vi "remoteControlDistance.vi"() -> ()   [LabVIEW 2019]
uses:
  <vilib>/ReMiSYS/ReMiSYS_WSCbot-XS/SubVI/XS_F710.ctl
  <vilib>/ReMiSYS/ReMiSYS_WSCbot-XS/SubVI/XS_stick.ctl
  <vilib>/ReMiSYS/ReMiSYS_WSCbot-XS/SubVI/XS_gamepadF710.lvclass
  <vilib>/Platform/TimedLoop/XDataNode/timing_clust.ctl
  <vilib>/Platform/TimedLoop/XDataNode/nitl_modes.ctl
  <vilib>/Platform/TimedLoop/XDataNode/wakeup.ctl
  <vilib>/platform/TimedLoop/XDataNode/XDataNode.xnode
  <vilib>/Platform/TimedLoop/XDataNode/XDNodeRunTimeDep.lvlib
  WSCbot_V3_Toolkit.lvlibp
panel:
  in  "Correction_distance(V)":dbl=1.5
  out "buttom array":bool[](array[boolean])
  out "Car move (cm)":dbl=-108.003392325
  out "Wheel move (cm)":dbl[](array[numeric])=[329.0260716, 275.9108976, 491.92183620000003, 545.0287023]
  out "F710 button info.leftStick":bool
  out "F710 button info.B":bool
  out "F710 button info.X":bool
  out "F710 button info.A":bool
  out "F710 button info.Y":bool
  out "F710 button info.RB":bool
  out "F710 button info.LB":bool
  out "ini":bool=TRUE
  out "reset":bool
  out "speed":dbl=800.0
  out "Error Out":errorcluster={"status"=FALSE, "code"=1073676418, "source"="VISA Close in XS_usbRawData (SubVI).vi:4400002->XS_gamepadF710.lvlib:XS_gamepadF710.lvclass:XS_grab.vi:4580001->remoteControlDistance.vi"}
  in  "Stop Button":bool
  in  "error in (no error)":errorcluster
  in  "INPUT S/N":string="U16N121E"
  in  "VISA resource name":refnum<visa-resource-name>="USB0::0x046D::0xC21F::145C9E1C::RAW"
  out "Stop Output":bool=TRUE
  out "StepmotorTarget(mm)":dbl=0.2
  out "AxisPosition":dbl
  out "SpeedArray":dbl[](array[numeric])
  out "F710":T1={"RT"=0, "LT"=0, "RightStick"=[{"X"=0.0, "Y"=1.0}], "LeftStick"=[{"X"=3.0, "Y"=0.0}], "Axis info"={"Left x-Axis"=3, "Left y-Axis"=0, "Right x-Axis"=0, "Righ y-Axis"=1, "LT"=0, "RT"=0}, "F710 button info"={"RB"=FALSE, "LB"=FALSE, "rightStick"=FALSE, "leftStick"=FALSE, "start"=FALSE, "back"=FALSE, "right"=FALSE, "left"=FALSE, "down"=FALSE, "up"=FALSE, "Y"=FALSE, "X"=FALSE, "B"=FALSE, "A"=FALSE, "LogiB"=FALSE}}
  in  "maxSpeed":dbl=800.0 format="%#_13g"
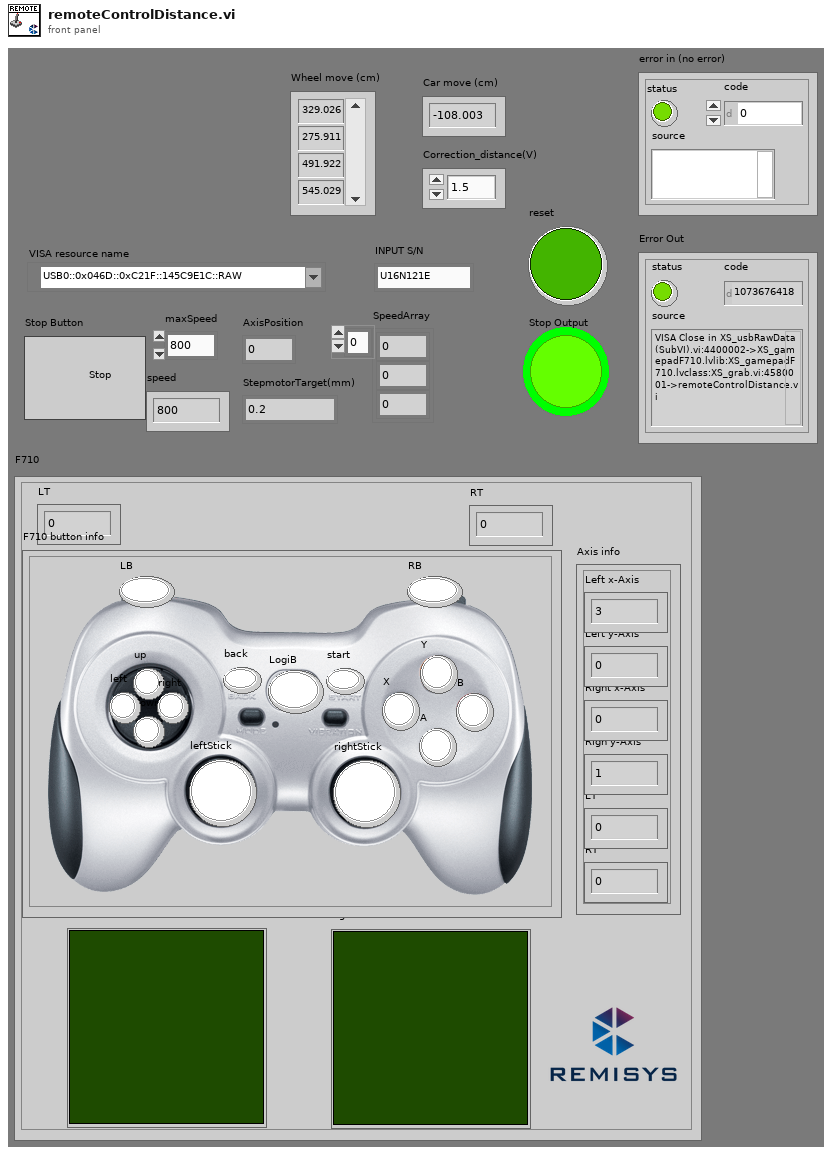
[diagram p1: front panel]
types:
  T1 = typedef "XS_F710.ctl" = cluster{"RT":u8, "LT":u8, "RightStick":T2, "LeftStick":T2, "Axis info":cluster{"Left x-Axis":i8, "Left y-Axis":i8, "Right x-Axis":i8, "Righ y-Axis":i8, "LT":u8, "RT":u8}, "F710 button info":cluster{"RB":bool, "LB":bool, "rightStick":bool, "leftStick":bool, "start":bool, "back":bool, "right":bool, "left":bool, "down":bool, "up":bool, "Y":bool, "X":bool, "B":bool, "A":bool, "LogiB":bool}}
  T2 = typedef "XS_stick.ctl" = cluster{"X":dbl, "Y":dbl}[]
  T3 = typedef "XDNodeRunTimeDep.lvlib/timing_clust.ctl" = cluster{"Expected End [f-1]":u64, "Actual End [f-1]":u64, "Finished Late? [f-1]":bool, "Expected End [i-1]":u64, "Actual End [i-1]":u64, "Finished Late? [i-1]":bool, "Expected Start [i]":u64, "Actual Start [i]":u64, "Expected Start [f]":u64, "Actual Start [f]":u64, "Source Name":string, "Structure Name":string, "Period":i64, "Deadline":i64, "Offset":i64, "Start":i64, "Priority":i32, "Timeout":i32, "Mode":T4, "Wakeup Reason":T5, "Error":errorcluster, "Source Type":string, "Secondary Source Type":string, "Global End Time":u64, "Global Start Time":u64, "Frame Duration":u64, "Iteration Duration":u64, "Assigned CPU":i32, "I/O Scan Engine Mode":u32}
  T4 = typedef "XDNodeRunTimeDep.lvlib/nitl_modes.ctl" = enum32{"No Change", "Process missed periods, maintain original phase", "Discard missed periods, maintain original phase", "Process missed periods, ignore original phase", "Discard missed periods, ignore original phase"}
  T5 = typedef "XDNodeRunTimeDep.lvlib/wakeup.ctl" = enum32{"Normal", "Aborted", "Asynchronous wakeup", "Timing source error", "Timed loop error", "Timeout"}
  T6 = enum16{"Right_up", "Right_down", "Left_down", "Left_up", "left", "right", "up", "down"}
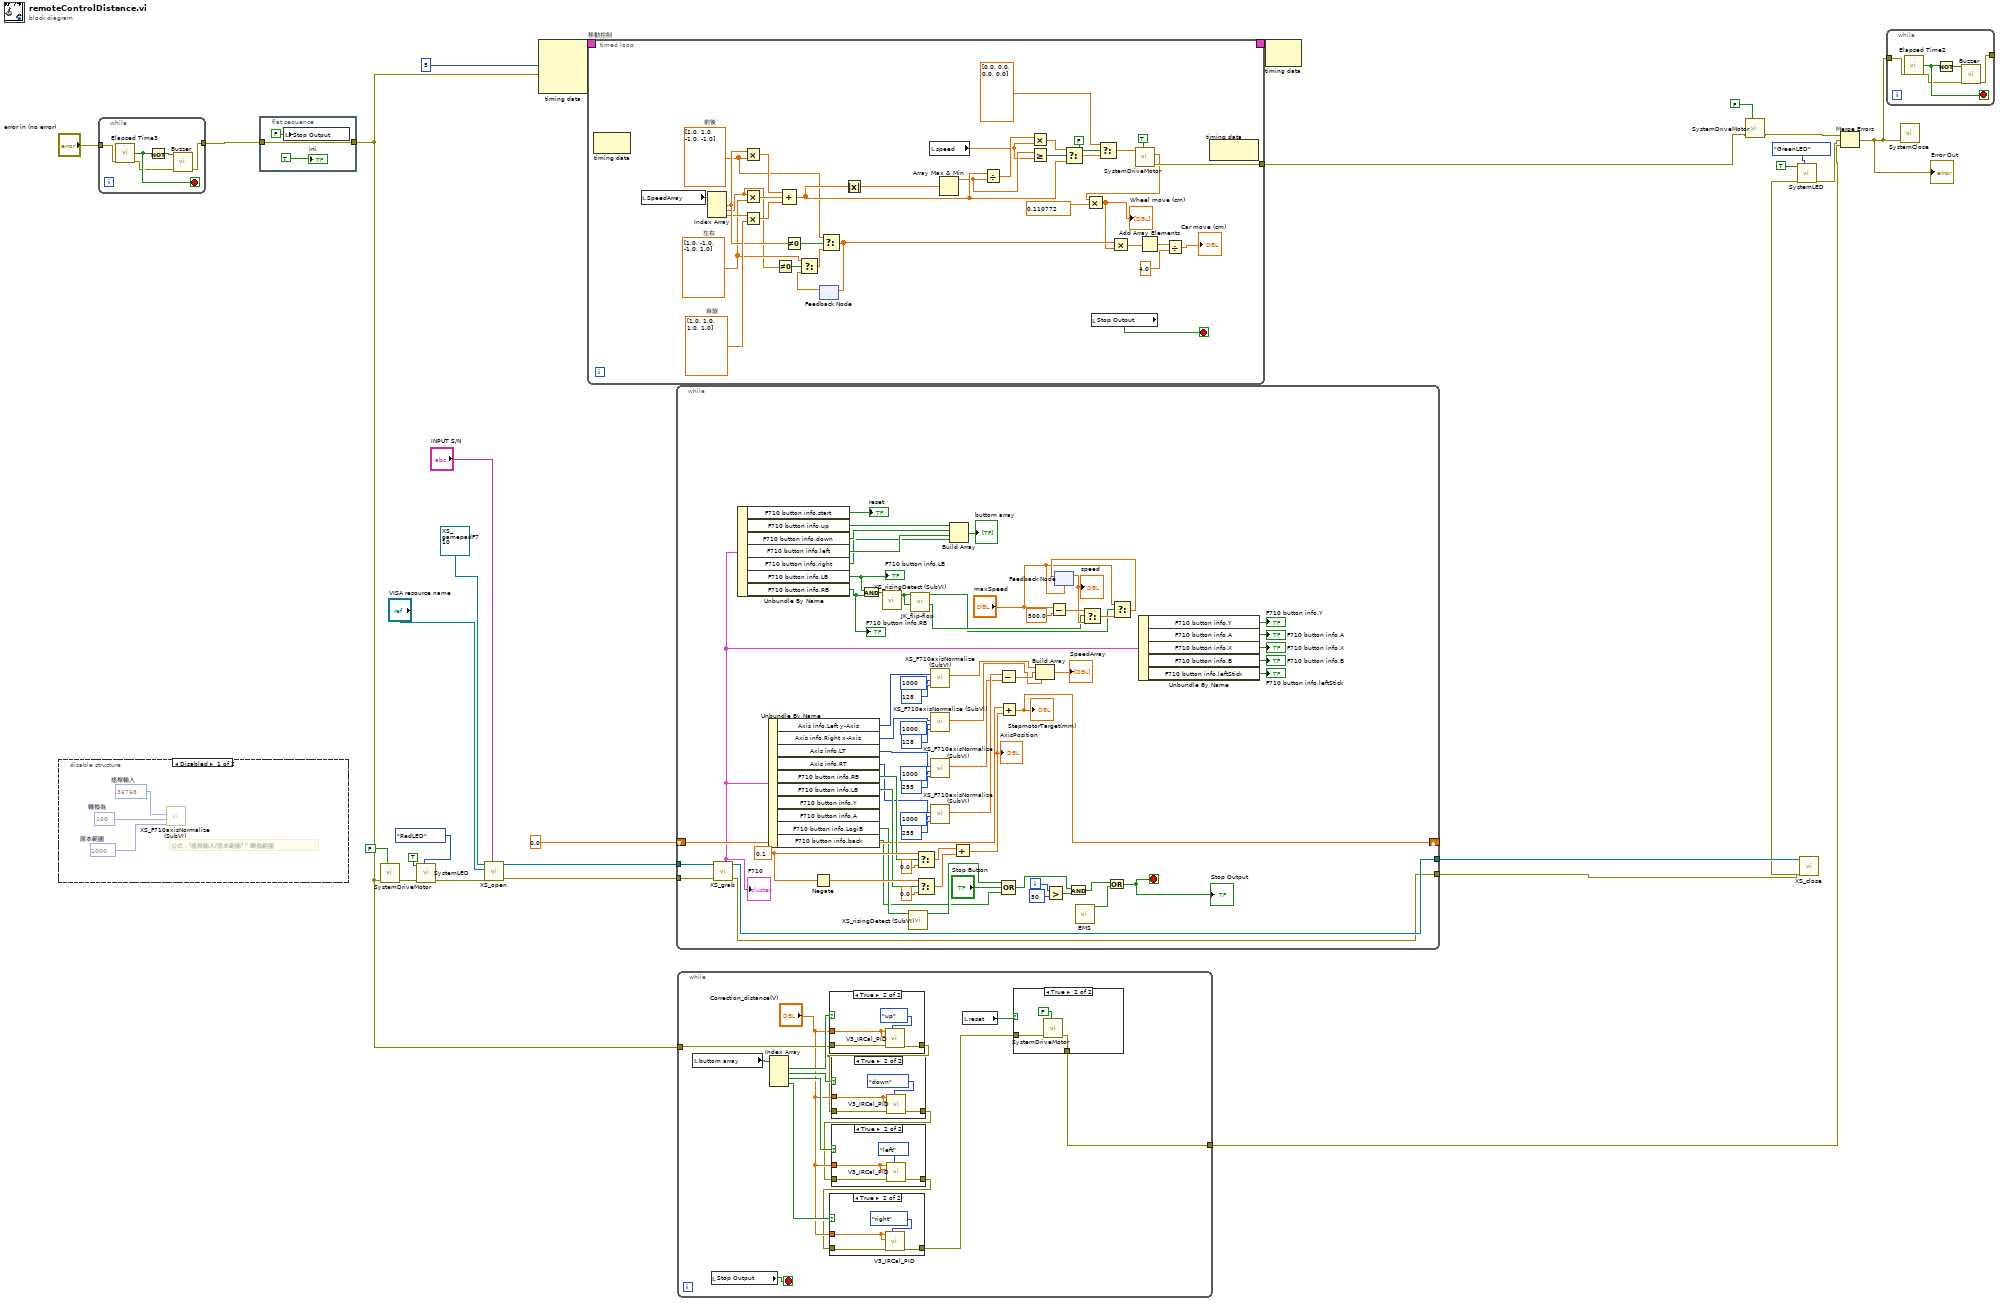
[diagram p0: block diagram]
diagram:
  n1 = disable-structure shown="Disabled" {
    frame Disabled {
      w29 = 1000  # 原本範圍
      w30 = 100  # 轉換為
      w31 = 36768  # 搖桿輸入
      # "公式：(搖桿輸入/原本範圍) * 轉換範圍"
      n2 = call <vilib>:"XS_F710axisNormalize (SubVI).vi"("rawRange"=w29, "normalizeTo"=w30, "axisInput"=w31) -> ()  [unwired: 8 in, 1 out]
    }
    frame Enabled {
    }
  }
  n3 = while {
    tunnel: "error in (no error)" -> [w34]
    tunnel: [w32] -> w11
    stop <- w36 stop-if-true
    n4 = call "Elapsed Time3"("error in (no error)"=w34) -> ("Time has Elapsed"=w36:bool, "error out"=w33:errorcluster)  [unwired: 11 in, 6 out]
    n5 = Not(x=w36) -> (.not. x?=w35:bool)
    n6 = call "Buzzer.vi"("error in"=w33, "Set"=w35) -> ("error out"=w32:errorcluster)  [unwired: 9 in]
  }
  n7 = flat-sequence {
    tunnel: [w38] -> w2
    tunnel: w11 -> [w38]
    frame #0 {
      n8 = local write "Stop Output"(FALSE ("Stop Output")) -> ()
      "ini" <- TRUE
    }
  }
  n9 = call "SystemDriveMotor.vi"("Enable?"=FALSE, "error in"=w2) -> ("error out"=w7:errorcluster)  [unwired: 8 in, 1 out]
  n10 = call "SystemLED.vi"("SelectColor"=enum16{"RedLED", "GreenLED", "YellowLED"}."RedLED", "error in"=w7, "Set"=TRUE) -> ("error out"=w18:errorcluster)  [unwired: 8 in]
  n11 = call <vilib>:"XS_open.vi"("INPUT S/N"="INPUT S/N", "error in (no error)"=w18, "VISA resource name"="VISA resource name", "gamepadF710 in"=refnum<class "XS_gamepadF710.lvclass"> refnum) -> ("error out"=w8:errorcluster, "gamepadF710 out"=w19:refnum<class "XS_gamepadF710.lvclass">)  [unwired: 6 in]
  n12 = node-c288(i64 5 ("Period"), w2) -> (w28:T3)  [unwired: 2 in]
  n13 = timed-loop "移動控制" {
    timing: w28 -> [_]
    timing-out: [_] -> w27
    tunnel: [w59] -> w5
    stop <- w64 stop-if-true
    w75 = dbl[] [1.0, 1.0, 1.0, 1.0]  # 自旋
    w49 = dbl[] [1.0, -1.0, -1.0, 1.0]  # 左右
    w50 = dbl[] [1.0, 1.0, -1.0, -1.0]  # 前後
    n14 = node-c288() -> ()  [unwired: 1 in, 1 out]
    n15 = local read "SpeedArray"() -> (w68:dbl[])
    n16 = Index Array(array=w68) -> (element #1=w53:dbl, element #2=w40:dbl, element #3=w51:dbl)  [unwired: 3 in]
    n17 = Multiply(x=w53, y=w50) -> (x*y=w74:dbl[])
    n18 = Multiply(x=w40, y=w49) -> (x*y=w73:dbl[])
    n19 = Multiply(x=w51, y=w75) -> (x*y=w72:dbl[])
    n20 = Not Equal To 0?(x=w40) -> (x != 0?=w52:bool)
    n21 = Compound Arithmetic op=ADD(w74, w73, w72) -> (w69:dbl[])
    n22 = Not Equal To 0?(x=w53) -> (x != 0?=w54:bool)
    n23 = feedback #1() -> (w47:dbl[])  [unwired: 1 in]
    n24 = Select(t=w49, s=w52, f=w47) -> (s? t:f=w48:dbl[])
    n25 = Select(t=w50, s=w54, f=w48) -> (s? t:f=w46:dbl[])
    n26 = feedback-in #1(w46) -> ()
    n27 = Absolute Value(x=w69) -> (abs(x)=w71:dbl[])
    n28 = local read "speed"() -> (w57:dbl)
    n29 = Array Max & Min(array=w71) -> (max value=w65:dbl)  [unwired: 3 out]
    n30 = Divide(x=w69, y=w65) -> (x/y=w67:dbl[])
    n31 = Multiply(x=w67, y=w57) -> (x*y=w66:dbl[])
    n32 = Greater Or Equal?(x=w65, y=w57) -> (x >= y?=w70:bool)
    n33 = Select(t=w66, s=w70, f=w69) -> (s? t:f=w63:dbl[])
    n34 = local read "Stop Output"() -> (w64:bool)
    n35 = Select(t=dbl[] [0.0, 0.0, 0.0, 0.0], s=FALSE, f=w63) -> (s? t:f=w61:dbl[])
    n36 = call "SystemDriveMotor.vi"("Enable?"=TRUE, "4xMotor(deg/s)"=w61) -> ("error out"=w59:errorcluster, "ENC (deg)"=w56:dbl[])  [unwired: 8 in]
    n37 = Multiply(x=w56, y=0.110772 ("Numeric")) -> (x*y=w45:dbl[])
    "Wheel move (cm)" <- w45
    n38 = Multiply(x=w46, y=w45) -> (x*y=w44:dbl[])
    n39 = Add Array Elements(numeric array=w44) -> (sum=w43:dbl)
    n40 = Divide(x=w43, y=4.0) -> (x/y=→"Car move (cm)":dbl)
    n41 = node-c288() -> ()  [unwired: 1 in, 1 out]
  }
  n42 = while {
    tunnel: w19 -> [w145]
    tunnel: [w144] -> w23
    tunnel: [w127] -> w22
    tunnel: w8 -> [w126]
    shift-right: [w122] -> _
    shift-left: 0.0 -> [w121]
    i -> [w119]
    stop <- w78 stop-if-true
    w128 = 0.1 ("t")
    n43 = call <vilib>:"XS_grab.vi"("error in (no error)"=w126, "gamepadF710 in"=w145) -> ("error out"=w127:errorcluster, "gamepadF710 out"=w144:refnum<class "XS_gamepadF710.lvclass">, "F710"=w91:T1)  [unwired: 6 in]
    "F710" <- w91
    n44 = Unbundle By Name(w91) -> ("F710 button info.start"=→"reset":bool, "F710 button info.up"=w85:bool, "F710 button info.down"=w84:bool, "F710 button info.left"=w83:bool, "F710 button info.right"=w82:bool, "F710 button info.LB"=w95:bool, "F710 button info.RB"=w96:bool)
    "F710 button info.LB" <- w95
    "F710 button info.RB" <- w96
    n45 = Unbundle By Name(w91) -> ("Axis info.Left y-Axis"=w112:i8, "Axis info.Right x-Axis"=w111:i8, "Axis info.LT"=w110:u8, "Axis info.RT"=w109:u8, "F710 button info.RB"=w125:bool, "F710 button info.LB"=w124:bool, "F710 button info.LogiB"=w115:bool, "F710 button info.back"=w114:bool)  [unwired: 2 out]
    n46 = Negate(x=w128) -> (-x=w129:dbl)
    n47 = And(x=w95, y=w96) -> (x .and. y?=w94:bool)
    n48 = call <vilib>:"XS_risingDetect (SubVI).vi"("y"=w94) -> ("Boolean"=w97:bool)  [unwired: 10 in]
    n49 = call <vilib>:"XS_risingDetect (SubVI).vi"("y"=w115) -> ("Boolean"=w120:bool)  [unwired: 10 in]
    n50 = call "JK_flip-flop.vi"("K"=w97, "J"=w97) -> ("Q"=w92:bool, "-Q"=w98:bool)  [unwired: 7 in]
    n51 = Select(t=w128, s=w125, f=0.0) -> (s? t:f=w130:dbl)
    n52 = Select(t=w129, s=w124, f=0.0) -> (s? t:f=w131:dbl)
    n53 = call <vilib>:"XS_F710axisNormalize (SubVI).vi"("rawRange"=128, "normalizeTo"=1000, "axisInput"=w112) -> ("NormalizedValue"=w135:dbl)  [unwired: 8 in]
    n54 = call <vilib>:"XS_F710axisNormalize (SubVI).vi"("rawRange"=128, "normalizeTo"=1000, "axisInput"=w111) -> ("NormalizedValue"=w107:dbl)  [unwired: 8 in]
    n55 = call <vilib>:"XS_F710axisNormalize (SubVI).vi"("rawRange"=255, "normalizeTo"=1000, "axisInput"=w110) -> ("NormalizedValue"=w105:dbl)  [unwired: 8 in]
    n56 = call <vilib>:"XS_F710axisNormalize (SubVI).vi"("rawRange"=255, "normalizeTo"=1000, "axisInput"=w109) -> ("NormalizedValue"=w106:dbl)  [unwired: 8 in]
    n57 = Build Array(w85, w84, w83, w82) -> (→"buttom array":bool[])
    n58 = Add(x=w130, y=w131) -> (x+y=w123:dbl)
    "AxisPosition" <- w123
    n59 = Subtract(x=w106, y=w105) -> (x-y=w108:dbl)
    n60 = Add(x=w121, y=w123) -> (x+y=w122:dbl)
    "StepmotorTarget(mm)" <- w122
    n61 = Compound Arithmetic op=OR(w120, "Stop Button", w114) -> (w116:bool)
    n62 = Build Array(w135, w108, w107) -> (→"SpeedArray":dbl[])
    n63 = Greater?(x=w119, y=50) -> (0:w117:bool)
    n64 = Subtract(x="maxSpeed", y=500.0) -> (x-y=w103:dbl)
    n65 = feedback #2("maxSpeed") -> (w100:dbl)
    "speed" <- w100
    n66 = And(x=w116, y=w117) -> (x .and. y?=w80:bool)
    n67 = call "EMS.vi"() -> ("EMS"=w79:bool)  [unwired: 10 in, 1 out]
    n68 = Select(t=w103, s=w98, f=w100) -> (s? t:f=w102:dbl)
    n69 = Or(x=w80, y=w79) -> (x .or. y?=w78:bool)
    "Stop Output" <- w78
    n70 = Select(t="maxSpeed", s=w92, f=w102) -> (s? t:f=w101:dbl)
    n71 = feedback-in #2(w101) -> ()
    n72 = Unbundle By Name(w91) -> ("F710 button info.Y"=→"F710 button info.Y":bool, "F710 button info.A"=→"F710 button info.A":bool, "F710 button info.X"=→"F710 button info.X":bool, "F710 button info.B"=→"F710 button info.B":bool, "F710 button info.leftStick"=→"F710 button info.leftStick":bool)
  }
  n73 = while {
    tunnel: w2 -> [w153]
    tunnel: [w146] -> w1
    stop <- w154 stop-if-true
    n74 = local read "buttom array"() -> (w159:bool[])
    n75 = local read "Stop Output"() -> (w154:bool)
    n76 = Index Array(array=w159) -> (element #1=w158:bool, element #2=w157:bool, element #3=w156:bool, element #4=w155:bool)  [unwired: 4 in]
    n77 = case shown="True" w158 {
      tunnel: w153 -> [w179 w182]
      tunnel: "Correction_distance(V)" -> [_ w181]
      tunnel: [w179 w180] -> w151
      frame False {
      }
      frame True {
        n78 = call "V3_IRCal_PID.vi"("Direction"=T6."up", "Error In"=w182, "Y_distance(V)"=w181, "X_distance(V)"=w181) -> ("Error Out"=w180:errorcluster)  [unwired: 6 in, 1 out]
      }
    }
    n79 = case shown="True" w157 {
      tunnel: w151 -> [w174 w177]
      tunnel: "Correction_distance(V)" -> [_ w176]
      tunnel: [w174 w175] -> w150
      frame False {
      }
      frame True {
        n80 = call "V3_IRCal_PID.vi"("Direction"=T6."down", "Error In"=w177, "Y_distance(V)"=w176, "X_distance(V)"=w176) -> ("Error Out"=w175:errorcluster)  [unwired: 6 in, 1 out]
      }
    }
    n81 = case shown="True" w156 {
      tunnel: w150 -> [w169 w172]
      tunnel: "Correction_distance(V)" -> [_ w171]
      tunnel: [w169 w170] -> w149
      frame False {
      }
      frame True {
        n82 = call "V3_IRCal_PID.vi"("Direction"=T6."left", "Error In"=w172, "Y_distance(V)"=w171, "X_distance(V)"=w171) -> ("Error Out"=w170:errorcluster)  [unwired: 6 in, 1 out]
      }
    }
    n83 = case shown="True" w155 {
      tunnel: w149 -> [w164 w167]
      tunnel: "Correction_distance(V)" -> [_ w166]
      tunnel: [w164 w165] -> w147
      frame False {
      }
      frame True {
        n84 = call "V3_IRCal_PID.vi"("Direction"=T6."right", "Error In"=w167, "Y_distance(V)"=w166, "X_distance(V)"=w166) -> ("Error Out"=w165:errorcluster)  [unwired: 6 in, 1 out]
      }
    }
    n85 = local read "reset"() -> (w148:bool)
    n86 = case shown="True" w148 {
      tunnel: w147 -> [w160 w162]
      tunnel: [w160 w161] -> w146
      frame False {
      }
      frame True {
        n87 = call "SystemDriveMotor.vi"("Enable?"=FALSE, "error in"=w162) -> ("error out"=w161:errorcluster)  [unwired: 8 in, 1 out]
      }
    }
  }
  n88 = node-c288(w27) -> ()  [unwired: 1 out]
  n89 = call "SystemDriveMotor.vi"("Enable?"=FALSE, "error in"=w5) -> ("error out"=w4:errorcluster)  [unwired: 8 in, 1 out]
  n90 = call <vilib>:"XS_close.vi"("error in (no error)"=w22, "gamepadF710 in"=w23) -> ("error out"=w15:errorcluster)  [unwired: 8 in, 1 out]
  n91 = call "SystemLED.vi"("SelectColor"=enum16{"RedLED", "GreenLED", "YellowLED"}."GreenLED", "error in"=w15, "Set"=TRUE) -> ("error out"=w9:errorcluster)  [unwired: 8 in]
  n92 = Merge Errors(w4, w9, w1) -> (w13:errorcluster)
  "Error Out" <- w13
  n93 = while {
    tunnel: w13 -> [w186]
    tunnel: [w184] -> _
    stop <- w188 stop-if-true
    n94 = call "Elapsed Time2"("error in (no error)"=w186) -> ("Time has Elapsed"=w188:bool, "error out"=w185:errorcluster)  [unwired: 11 in, 6 out]
    n95 = Not(x=w188) -> (.not. x?=w187:bool)
    n96 = call "Buzzer.vi"("error in"=w185, "Set"=w187) -> ("error out"=w184:errorcluster)  [unwired: 9 in]
  }
  n97 = call "SystemClose.vi"("error in"=w13) -> ()  [unwired: 2 in, 1 out]
